vi "Create Pattern Script - Rd Data Frame.vi"(8 "error in (no error)":errorcluster, 10 "FRM Data":T1 {"Addr" format="%x"; "Data" format="%x"}, 11 "SPI 4W Pattern Creator in":refnum<class "SPI 4W Pattern Creator.lvclass">) -> (0 "error out":errorcluster, 2 "String":string, 3 "SPI 4W Pattern Creator out":refnum<class "SPI 4W Pattern Creator.lvclass">)   [LabVIEW 2018, in "SPI 4W Pattern Creator.lvlib" / "SPI 4W Pattern Creator.lvclass"]
uses:
  SPI 4W Pattern Creator.lvclass
  Ctls/Frame Data - SPI_3W.ctl
  Ctls/RW Options.ctl
  Protocols/SPI Root Pattern Creator.lvlibp/Plugins/SouceCode/SPI_Pattern Creator/SPI Root/Special Frame Type.ctl
  Protocols/SPI Root Pattern Creator.lvlibp/Plugins/SouceCode/SPI_Pattern Creator/SPI Root/SPI Root Pattern Creator.lvclass
  C:/P4 Workspace/PC Client/Solutions/5g_eap/trunk/1.0/HiSi5GmmWave/Pattern_Gen_Tool/Plugins/Protocols/SPI Root Pattern Creator.lvlibp/Plugins/SouceCode/SPI_Pattern Creator/SPI Root/SPI Root Pattern Creator.lvclass
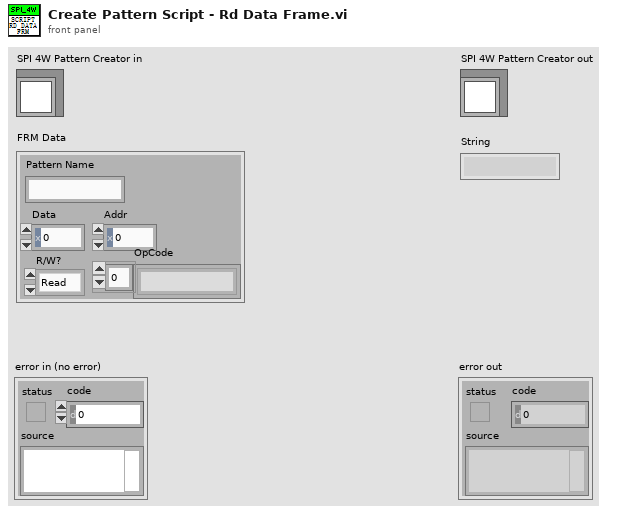
[diagram p1: front panel]
types:
  T1 = typedef "Frame Data - SPI_3W.ctl" = cluster{"Pattern Name":string, "Data":u16, "Addr":u16, "OpCode":string[], "R/W?":T2}
  T2 = typedef "RW Options.ctl" = enum16{"Read", "Write", "R/W"}
  T3 = typedef "SPI Root Pattern Creator.lvlibp/SPI Root Pattern Creator.lvclass/Special Frame Type.ctl" = enum16{"SPI 4W FRM Start", "SPI 4W Wait", "SPI 4W FRM End", "SPI 4W Write Cmd", "SPI Rd Collect Cmd", "SPI Rd Value Cmd", "SPI 3W FRM Start", "SPI 3W Write Cmd", "SPI 3W FRM End", "SPI 3W Wait", "SPI 3W Rd Cmd"}
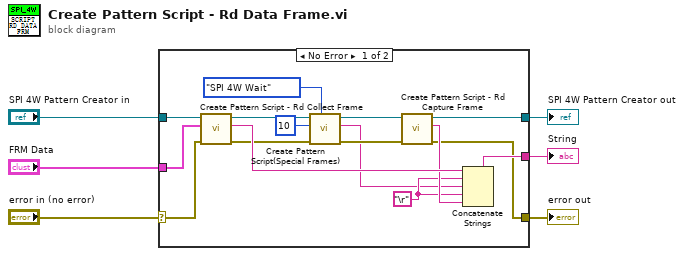
[diagram p0: block diagram]
diagram:
  n1 = case shown="No Error" "error in (no error)" {
    selector: "error in (no error)" -> [w20 w24]
    tunnel: "SPI 4W Pattern Creator in" -> [w22 w23]
    tunnel: "FRM Data" -> [w21 _]
    tunnel: [w16 _] -> w3
    tunnel: [w15 w23] -> w2
    tunnel: [w14 w24] -> w1
    frame No Error {
      w17 = "\r"
      n2 = call-dynamic "Create Pattern Script - Rd Collect Frame.vi"("error in (no error)"=w20, "FRM Data"=w21, "SPI 4W Pattern Creator in"=w22) -> ("error out"=w11:errorcluster, "String"=w19:string, "SPI 4W Pattern Creator out"=w13:refnum<class "SPI 4W Pattern Creator.lvclass">)  [unwired: 6 in]
      n3 = call "Create Pattern Script(Special Frames).vi"("Special Frame Type"=Special_Frame_Type."SPI 4W Wait", "error in (no error)"=w11, "Num of Timeset"=u32 10, "SPI Root Pattern Creator in"=w13) -> ("error out"=w9:errorcluster, "String out"=w8:string, "SPI Root Pattern Creator out"=w10:refnum<class "SPI 4W Pattern Creator.lvclass">)  [unwired: 5 in]
      n4 = call-dynamic "Create Pattern Script - Rd Capture Frame.vi"("error in (no error)"=w9, "SPI 4W Pattern Creator in"=w10) -> ("error out"=w14:errorcluster, "String"=w18:string, "SPI 4W Pattern Creator out"=w15:refnum<class "SPI 4W Pattern Creator.lvclass">)  [unwired: 7 in]
      n5 = Concatenate Strings(w19, w17, w8, w17, w18) -> (w16:string)
    }
    frame Error {
    }
  }
  "error out" <- w1
  "SPI 4W Pattern Creator out" <- w2
  "String" <- w3
